vi "analog_input_tool.vi"() -> ()   [LabVIEW 2013, in "Analog_Input.lvclass"]
uses:
  Analog_Input.lvclass
  <vilib>/Utility/error.llb/DialogType.ctl
  <vilib>/DAQmx/read.llb/DAQmx Read (Analog 1D Wfm NChan 1Samp).vi
  <vilib>/DAQmx/create/channels.llb/DAQmx Create Channel (AI-Voltage-Basic).vi
  <vilib>/DAQmx/configure/timing.llb/DAQmx Timing (Sample Clock).vi
  Globals.vi
  <vilib>/DAQmx/miscellaneous.llb/DAQmx Fill In Error Info.vi
  <vilib>/Utility/file.llb/Write To Spreadsheet File (string).vi
panel:
  out "Coupling chart":dbl(graph)
  in  "Save Data?":bool
  in  "sample rate":dbl=5.0
  in  "error in":errorcluster
  in  "physical channels":tag="PXI1Slot7/ai0:2"
  out "Wattage chart":waveform(dbl)[](graph)=[{"t0"=timestamp(3447155546.350586 s since 1904-01-01), "dt"=0.2, "Y"=[8.096373353174213], "attributes"=variant("NI_ChannelName"=variant(string "PXI1Slot7/ai0"), "NI_UnitDescription"=variant(string "Volts"))}, {"t0"=timestamp(3447155546.350597 s since 1904-01-01), "dt"=0.2, "Y"=[0.029310863509207197], "attributes"=variant("NI_ChannelName"=variant(string "PXI1Slot7/ai1"), "NI_UnitDescription"=variant(string "Volts"))}, {"t0"=timestamp(3447155546.350608 s since 1904-01-01), "dt"=0.2, "Y"=[8.062512384255392], "attributes"=variant("NI_ChannelName"=variant(string "PXI1Slot7/ai2"), "NI_UnitDescription"=variant(string "Volts"))}]
  in  "location":string[](array[string])=["out of SHG crystal", "before fiber", "after fiber"]
  out "voltage":dbl[](array[numeric])=[2.1084305607224514, 0.01980463750622108, 1.6125024768510783]
  out "watts":dbl[](array[numeric])=[8.096373353174213, 0.029310863509207197, 8.062512384255392] format="%#_4g"
  in  "scaling":dbl[](array[numeric])=[3.84, 1.48, 5.0]
  in  "stop (F)":bool=TRUE
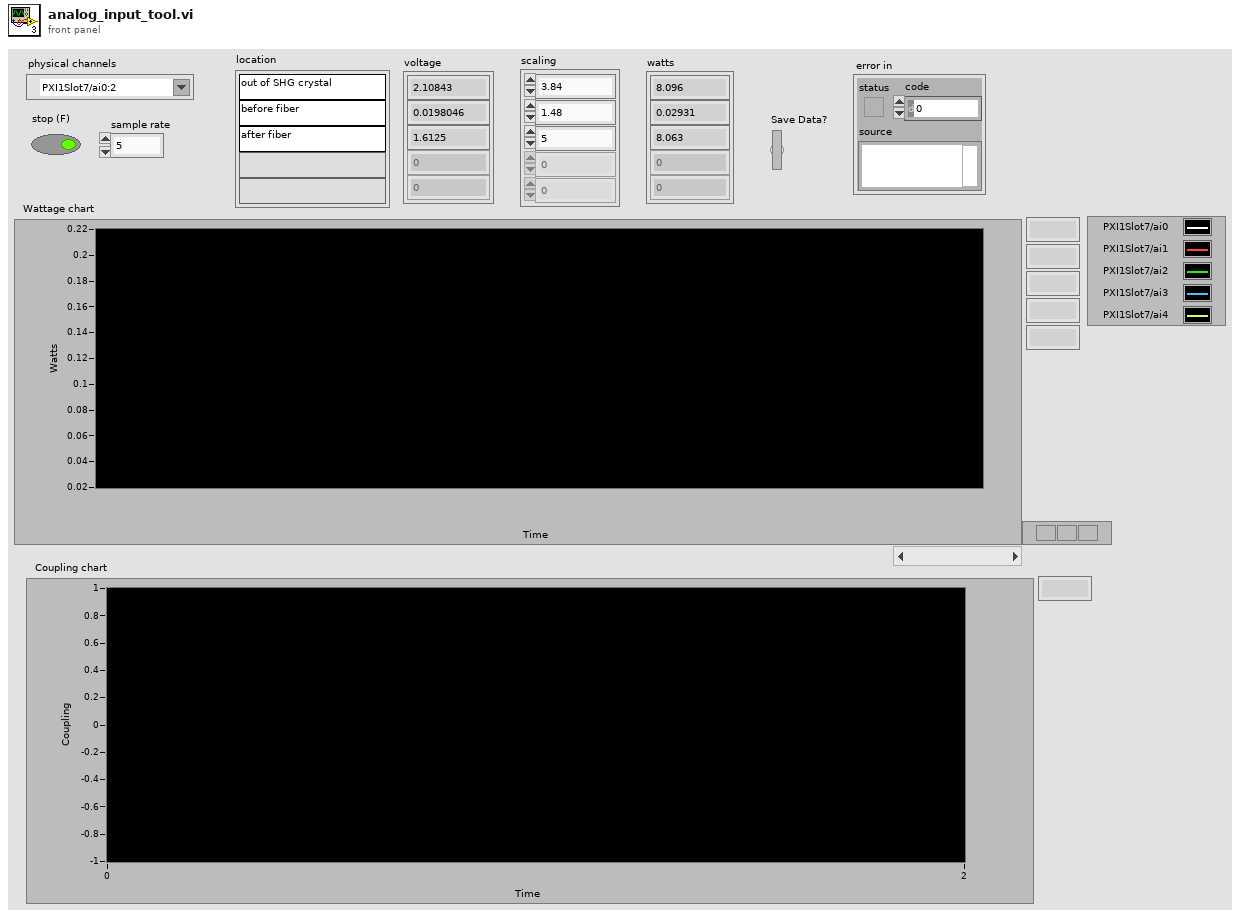
[diagram p1: front panel]
types:
  T1 = typedef "DialogType.ctl" = u16
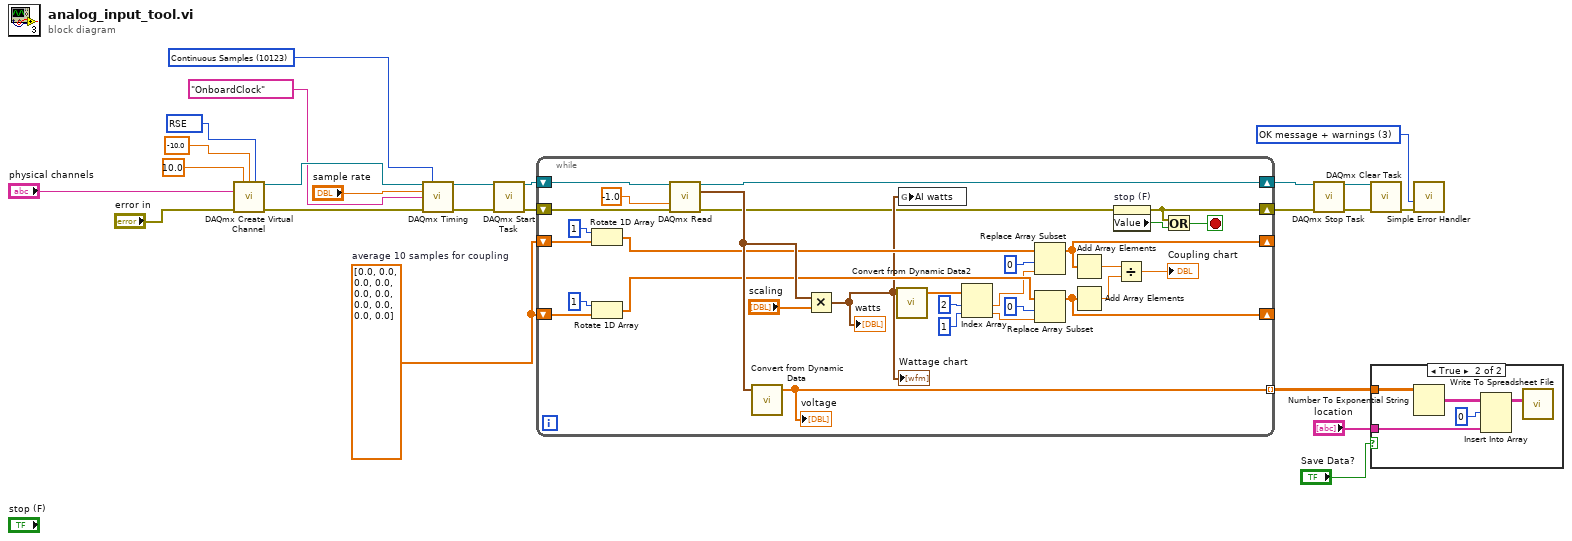
[diagram p0: block diagram]
diagram:
  w1 = dbl[] [0.0, 0.0, 0.0, 0.0, 0.0, 0.0, 0.0, 0.0, 0.0, 0.0]  # average 10 samples for coupling
  w9 = T1 3 items=["no dialog", "OK message", "continue or stop message", "OK message + warnings", "continue/stop + warnings"] ("type of dialog (OK msg:1)")
  w14 = 10123 items=["Finite Samples"=10178, "Continuous Samples"=10123, "Hardware Timed Single Point"=12522] ("sample mode")
  w23 = 10083 items=["default"=-1, "RSE"=10083, "NRSE"=10078, "Differential"=10106, "Pseudodifferential"=12529] ("input terminal configuration")
  n1 = call-poly <vilib>:"DAQmx Create Virtual Channel.vi"("maximum value"=10.0, "minimum value"=-10.0, "input terminal configuration"=w23, "physical channels"="physical channels", "error in"="error in") -> ("task out"=w16:refnum<k21>, "error out"=w15:errorcluster)  [unwired: 9 in]
  n2 = call-poly <vilib>:"DAQmx Timing.vi"("task/channels in"=w16, "sample mode"=w14, "rate"="sample rate", "source"=tag "OnboardClock", "error in"=w15) -> ("task out"=w10:refnum<k21>, "error out"=w11:errorcluster)  [unwired: 9 in]
  n3 = call <vilib>:"DAQmx Start Task.vi"("task/channels in"=w10, "error in"=w11) -> ("task out"=w18:refnum<k21>, "error out"=w19:errorcluster)  [unwired: 12 in]
  n4 = while {
    shift-right: [w46] -> w8
    shift-left: w19 -> [w53]
    shift-right: [w52] -> w17
    shift-left: w18 -> [w54]
    tunnel: [w50] -> w5 mode=indexing
    shift-right: [w30] -> _
    shift-left: w1 -> [w39]
    shift-right: [w29] -> _
    shift-left: w1 -> [w31]
    stop <- w49 stop-if-true
    n5 = Rotate 1D Array(1:w39, 2:1 ("n")) -> (0:w38:dbl[])
    n6 = Rotate 1D Array(1:w31, 2:1 ("n")) -> (0:w41:dbl[])
    n7 = call-poly <vilib>:"DAQmx Read.vi"("task/channels in"=w54, "timeout"=-1.0, "error in"=w53) -> ("task out"=w52:refnum<k21>, "data"=w45:waveform(dbl)[], "error out"=w25:errorcluster)  [unwired: 10 in]
    n8 = call "Convert from Dynamic Data"("Dynamic Data Type"=w45) -> ("Array"=w50:dbl[])  [unwired: 3 in]
    "voltage" <- w50
    n9 = Multiply(x=w45, y="scaling") -> (x*y=w26:waveform(dbl)[])
    "watts" <- w26
    "Wattage chart" <- w26
    n10 = call "Convert from Dynamic Data2"("Dynamic Data Type"=w26) -> ("Array"=w40:dbl[])  [unwired: 3 in]
    n11 = global write "Globals.vi" "AI watts"(w26) -> ()
    n12 = Index Array(array=w40, index #1=2 ("index"), index #2=1 ("index")) -> (element #1=w35:dbl, element #2=w32:dbl)
    n13 = Replace Array Subset(array=w38, new element=w35, index=0) -> (w30:dbl[])
    n14 = Replace Array Subset(array=w41, new element=w32, index=0) -> (w29:dbl[])
    n15 = Add Array Elements(numeric array=w30) -> (sum=w27:dbl)
    n16 = Add Array Elements(numeric array=w29) -> (sum=w28:dbl)
    n17 = property on="stop (F)" class="Bool (strict)"(error in=w25) -> (error out=w46:errorcluster, "Value"=w47:bool)  [unwired: 1 in, 1 out]
    n18 = Divide(x=w27, y=w28) -> (x/y=→"Coupling chart":dbl)
    n19 = Or(x=w46, y=w47) -> (x .or. y?=w49:bool)
  }
  n20 = call <vilib>:"DAQmx Stop Task.vi"("task/channels in"=w17, "error in"=w8) -> ("task out"=w20:refnum<k21>, "error out"=w21:errorcluster)  [unwired: 12 in]
  n21 = call <vilib>:"DAQmx Clear Task.vi"("task in"=w20, "error in"=w21) -> ("error out"=w7:errorcluster)  [unwired: 13 in]
  n22 = case shown="True" "Save Data?" {
    tunnel: "location" -> [_ w59]
    tunnel: w5 -> [_ w57]
    frame False {
    }
    frame True {
      n23 = Number To Exponential String(number=w57) -> (E-format string=w56:string[][])  [unwired: 3 in]
      n24 = Insert Into Array(array=w56, index (row)=0, new element=w59) -> (w55:string[][])  [unwired: 1 in]
      n25 = call-poly <vilib>:"Write To Spreadsheet File.vi"("2D data"=w55) -> ()  [unwired: 7 in, 1 out]
    }
  }
  n26 = call <vilib>:"Simple Error Handler.vi"("type of dialog (OK msg:1)"=w9, "error in (no error)"=w7) -> ()  [unwired: 3 in, 5 out]
